vi "Get timestamp from MS filename.vi"(0 "Filename":string) -> (1 "Subject":i32, 2 "Sample age /hours":dbl, 3 "Measurement Time Stamp":timestamp, 4 "Sample Time Stamp":timestamp)   [LabVIEW 2015]
uses:
  <vilib>/Utility/miscctls.llb/LVDateTimeRec.ctl
panel:
  out "Sample Year":i32
  out "Sample Month":i32
  out "Sample m":i32
  out "Sample h":i32
  out "Sample Day":i32
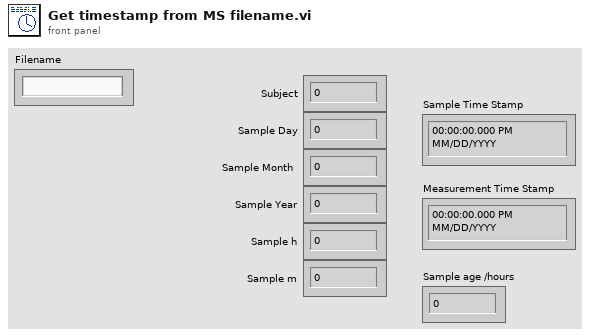
[diagram p1: front panel]
types:
  T1 = typedef "LVDateTimeRec.ctl" = cluster{"fractional second":dbl, "second":i32, "minute":i32, "hour":i32, "day of month":i32, "month":i32, "year":i32, "day of week":i32, "day of year":i32, "DST":i32}
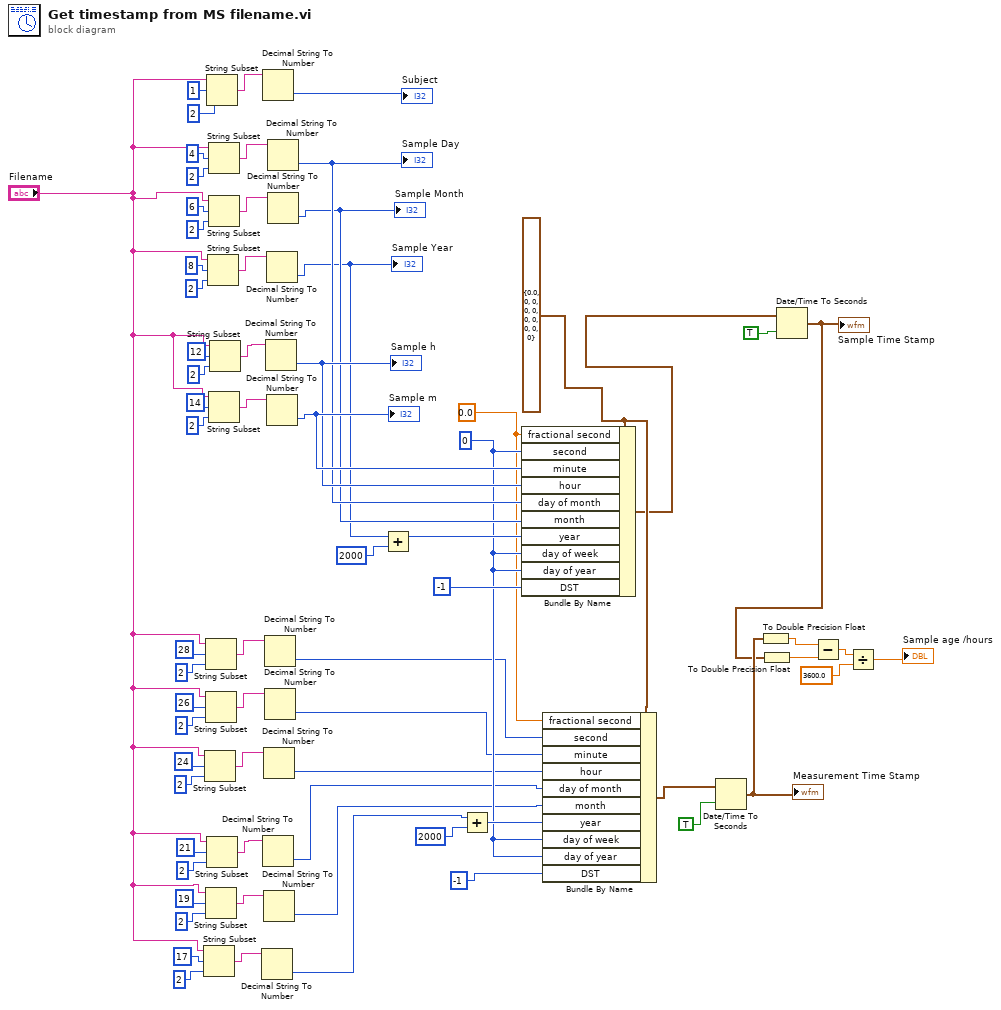
[diagram p0: block diagram]
diagram:
  w19 = T1 {"fractional second"=0.0, "second"=0, "minute"=0, "hour"=0, "day of month"=0, "month"=0, "year"=0, "day of week"=0, "day of year"=0, "DST"=0} ("date time rec")
  w18 = 0
  w17 = 0.0
  n1 = String Subset(string="Filename", offset (0)=17, length (rest)=2) -> (substring=w24:string)
  n2 = String Subset(string="Filename", offset (0)=24, length (rest)=2) -> (substring=w27:string)
  n3 = String Subset(string="Filename", offset (0)=28, length (rest)=2) -> (substring=w35:string)
  n4 = String Subset(string="Filename", offset (0)=26, length (rest)=2) -> (substring=w28:string)
  n5 = String Subset(string="Filename", offset (0)=19, length (rest)=2) -> (substring=w33:string)
  n6 = String Subset(string="Filename", offset (0)=1, length (rest)=2) -> (substring=w60:string)
  n7 = String Subset(string="Filename", offset (0)=21, length (rest)=2) -> (substring=w34:string)
  n8 = String Subset(string="Filename", offset (0)=8, length (rest)=2) -> (substring=w51:string)
  n9 = String Subset(string="Filename", offset (0)=4, length (rest)=2) -> (substring=w59:string)
  n10 = String Subset(string="Filename", offset (0)=6, length (rest)=2) -> (substring=w52:string)
  n11 = String Subset(string="Filename", offset (0)=14, length (rest)=2) -> (substring=w57:string)
  n12 = String Subset(string="Filename", offset (0)=12, length (rest)=2) -> (substring=w58:string)
  n13 = Decimal String To Number(string=w24) -> (number=w11:i32)  [unwired: 2 in, 1 out]
  n14 = Decimal String To Number(string=w60) -> (number=→"Subject":i32)  [unwired: 2 in, 1 out]
  n15 = Decimal String To Number(string=w34) -> (number=w13:i32)  [unwired: 2 in, 1 out]
  n16 = Decimal String To Number(string=w27) -> (number=w14:i32)  [unwired: 2 in, 1 out]
  n17 = Decimal String To Number(string=w33) -> (number=w12:i32)  [unwired: 2 in, 1 out]
  n18 = Decimal String To Number(string=w35) -> (number=w16:i32)  [unwired: 2 in, 1 out]
  n19 = Decimal String To Number(string=w28) -> (number=w15:i32)  [unwired: 2 in, 1 out]
  n20 = Decimal String To Number(string=w58) -> (number=w49:i32)  [unwired: 2 in, 1 out]
  "Sample h" <- w49
  n21 = Decimal String To Number(string=w51) -> (number=w44:i32)  [unwired: 2 in, 1 out]
  "Sample Year" <- w44
  n22 = Decimal String To Number(string=w57) -> (number=w50:i32)  [unwired: 2 in, 1 out]
  "Sample m" <- w50
  n23 = Decimal String To Number(string=w59) -> (number=w48:i32)  [unwired: 2 in, 1 out]
  "Sample Day" <- w48
  n24 = Decimal String To Number(string=w52) -> (number=w47:i32)  [unwired: 2 in, 1 out]
  "Sample Month" <- w47
  n25 = Add(x=w44, y=2000) -> (x+y=w43:i32)
  n26 = Add(x=w11, y=2000) -> (x+y=w20:i32)
  n27 = Bundle By Name(cluster=w19, "fractional second"=w17, "second"=w18, "minute"=w50, "hour"=w49, "day of month"=w48, "month"=w47, "year"=w43, "day of week"=w18, "day of year"=w18, "DST"=-1) -> (w8:T1)
  n28 = Bundle By Name(cluster=w19, "fractional second"=w17, "second"=w16, "minute"=w15, "hour"=w14, "day of month"=w13, "month"=w12, "year"=w20, "day of week"=w18, "day of year"=w18, "DST"=-1) -> (w9:T1)
  n29 = Date/Time To Seconds(1:TRUE, 2:w9) -> (0:w5:timestamp)
  "Measurement Time Stamp" <- w5
  n30 = To Double Precision Float(number=w5) -> (double precision float=w3:dbl)
  n31 = Date/Time To Seconds(1:TRUE, 2:w8) -> (0:w4:timestamp)
  "Sample Time Stamp" <- w4
  n32 = To Double Precision Float(number=w4) -> (double precision float=w2:dbl)
  n33 = Subtract(x=w3, y=w2) -> (x-y=w1:dbl)
  n34 = Divide(x=w1, y=3600.0) -> (x/y=→"Sample age /hours":dbl)
